vi "PlaneFromPoints.vi"(3 "Points":T1) -> (0 "D":dbl, 1 "Plane":cluster{"A":dbl, "B":dbl, "C":dbl})   [LabVIEW 2014]
uses:
  <vilib>/Analysis/NI_AALPro.lvlib
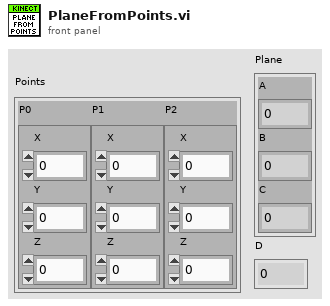
[diagram p1: front panel]
types:
  T1 = cluster{"P0":cluster{"X":dbl, "Y":dbl, "Z":dbl}, "P1":cluster{"X":dbl, "Y":dbl, "Z":dbl}, "P2":cluster{"X":dbl, "Y":dbl, "Z":dbl}}
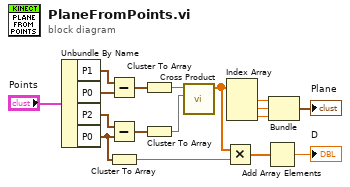
[diagram p0: block diagram]
diagram:
  n1 = Unbundle By Name("Points") -> ("P1"=w16:cluster{"X":dbl, "Y":dbl, "Z":dbl}, "P0"=w15:cluster{"X":dbl, "Y":dbl, "Z":dbl}, "P2"=w14:cluster{"X":dbl, "Y":dbl, "Z":dbl}, "P0"=w9:cluster{"X":dbl, "Y":dbl, "Z":dbl})
  n2 = Subtract(x=w16, y=w15) -> (x-y=w13:cluster{"X":dbl, "Y":dbl, "Z":dbl})
  n3 = Subtract(x=w14, y=w9) -> (x-y=w12:cluster{"X":dbl, "Y":dbl, "Z":dbl})
  n4 = Cluster To Array(cluster=w9) -> (array=w8:dbl[])
  n5 = Cluster To Array(cluster=w13) -> (array=w10:dbl[])
  n6 = Cluster To Array(cluster=w12) -> (array=w11:dbl[])
  n7 = call <vilib>:"Cross Product.vi"("B Vector"=w11, "A Vector"=w10) -> ("Cross Product"=w6:dbl[])  [unwired: 8 in, 1 out]
  n8 = Multiply(x=w6, y=w8) -> (x*y=w7:dbl[])
  n9 = Index Array(array=w6) -> (element #1=w4:dbl, element #2=w5:dbl, element #3=w3:dbl)  [unwired: 3 in]
  n10 = Add Array Elements(numeric array=w7) -> (sum=→"D":dbl)
  n11 = Bundle(w4, w5, w3) -> (→"Plane":cluster{dbl, dbl, dbl})  [unwired: 1 in]
